vi "Gettag.vi"(0 "TagName":string="caca", 1 "XML":string="aaaa\n<caca noseque=nosecuanto>\nmás cosas\n</caca>\ndfsdf") -> (2 "AfterTag":string, 3 "InsideTag":string, 4 "BeforeTag":string="aaaa\n<caca noseque=nosecuanto>\nmás cosas\n</caca>\ndfsdf", 5 "Found?":bool)   [LabVIEW 2010]
panel:
  out "temp":string
  out "Inside":string
  out "N":i32=1
  # "This vi gets the contents of a tag and the strings after and before"
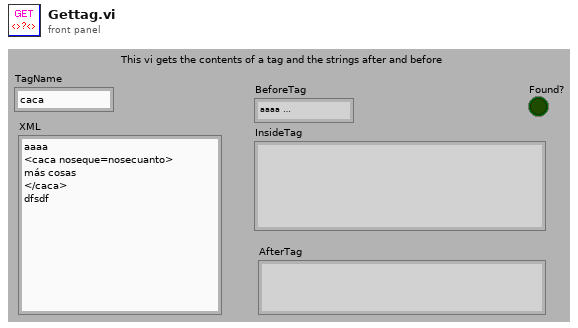
[diagram p1: front panel]
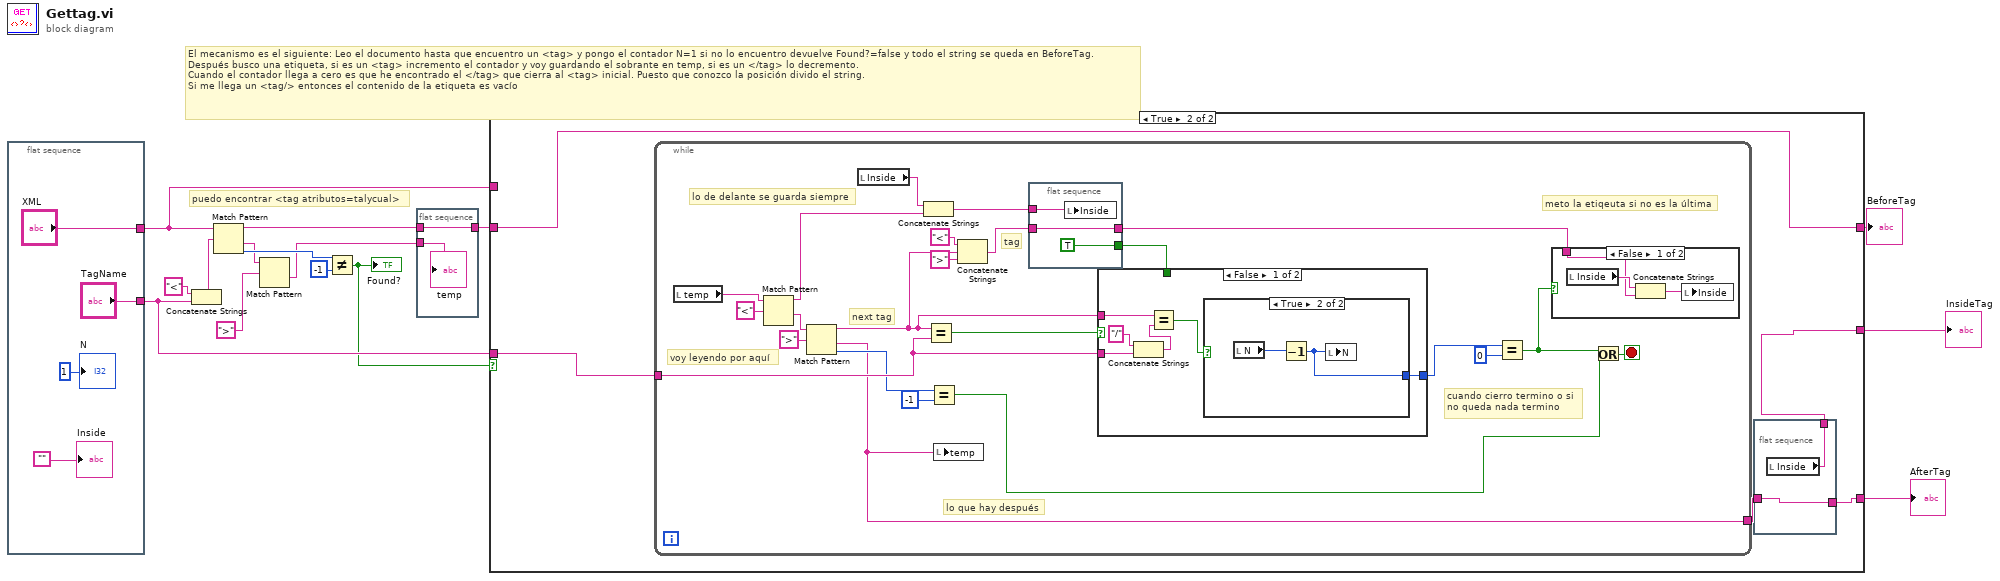
[diagram p0: block diagram]
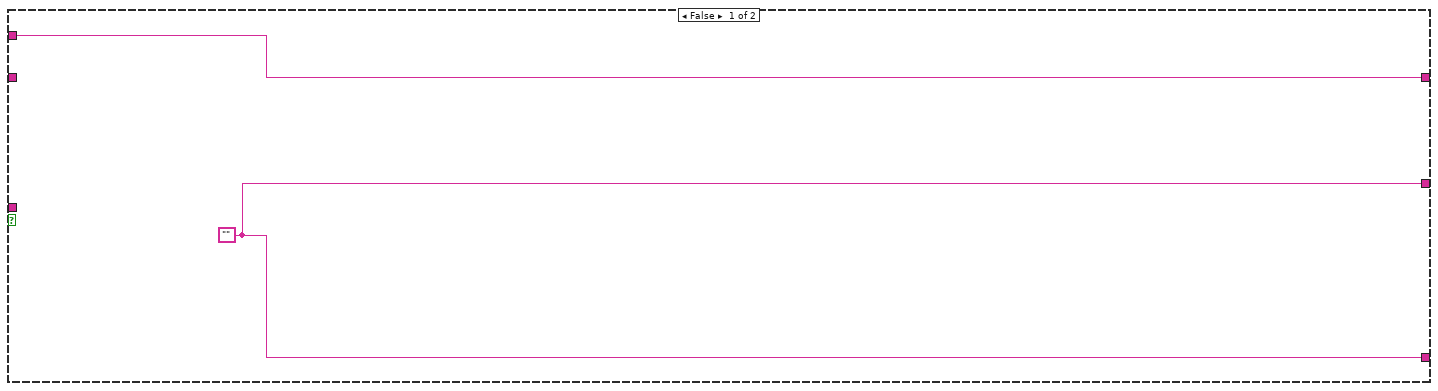
[diagram p2: hidden frame]
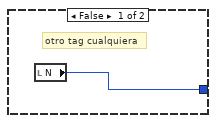
[diagram p4: hidden frame]
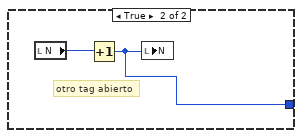
[diagram p5: hidden frame]
diagram:
  # "puedo encontrar <tag atributos=talycual>"
  # "El mecanismo es el siguiente: Leo el documento hasta que encuentro un <tag> y pongo el contador N=1 si no lo encuentro devuelve Found?=false y todo el string se queda en BeforeTag.\nDespués busco una etiqueta, si es un <tag> incremento el contador y voy guardando el sobrante en temp, si es un </tag> lo decremento.\nCuando el contador llega a cero es que he encontrado el </tag> que cierra al <tag> inicial. Puesto que conozco la posición divido el string.\nSi me llega un <tag/> entonces el contenido de la etiqueta es vacío"
  n1 = flat-sequence {
    tunnel: ["XML"] -> w11
    tunnel: ["TagName"] -> w7
    frame #0 {
      "N" <- 1
      "Inside" <- ""
    }
  }
  n2 = Concatenate Strings("<" ("string"), w7) -> (w8:string)
  n3 = Match Pattern(string=w11, regular expression=w8) -> (before substring=w5:string, after substring=w3:string, offset past match=w14:i32)  [unwired: 1 in, 1 out]
  n4 = Match Pattern(string=w3, regular expression=">" ("string")) -> (after substring=w1:string)  [unwired: 1 in, 3 out]
  n5 = Not Equal?(x=w14, y=-1) -> (x != y?=w6:bool)
  "Found?" <- w6
  n6 = flat-sequence {
    tunnel: w1 -> [w21]
    tunnel: w5 -> [w20]
    tunnel: [w20] -> w4
    frame #0 {
      "temp" <- w21
    }
  }
  n7 = case shown="True" w6 {
    tunnel: [w23 w27] -> w12
    tunnel: w4 -> [_ w27]
    tunnel: w11 -> [w23 _]
    tunnel: [w22 w24] -> w10
    tunnel: [w22 w26] -> w9
    tunnel: w7 -> [_ w28]
    frame False {
      w22 = ""
    }
    frame True {
      n8 = while {
        tunnel: w28 -> [w49]
        tunnel: [w39] -> w25
        stop <- w44 stop-if-true
        # "meto la etiqeuta si no es la última"
        # "lo de delante se guarda siempre"
        # "tag"
        # "lo que hay después"
        # "cuando cierro termino o si\nno queda nada termino"
        # "voy leyendo por aquí"
        # "next tag"
        n9 = local read "temp"() -> (w47:string)
        n10 = Match Pattern(string=w47, regular expression="<") -> (before substring=w36:string, after substring=w53:string)  [unwired: 1 in, 2 out]
        n11 = Match Pattern(string=w53, regular expression=">") -> (before substring=w42:string, after substring=w39:string, offset past match=w46:i32)  [unwired: 1 in, 1 out]
        n12 = local read "Inside"() -> (w37:string)
        n13 = Concatenate Strings(w37, w36) -> (w43:string)
        n14 = Equal?(x=w42, y=w49) -> (x = y?=w51:bool)
        n15 = Equal?(x=w46, y=-1) -> (x = y?=w34:bool)
        n16 = local write "temp"(w39) -> ()
        n17 = Concatenate Strings("<" ("before substring"), w42, ">" ("string")) -> (w38:string)
        n18 = flat-sequence {
          tunnel: w43 -> [w59]
          tunnel: w38 -> [w58]
          tunnel: [w58] -> w32
          tunnel: [TRUE] -> w31
          frame #0 {
            n19 = local write "Inside"(w59) -> ()
          }
        }
        n20 = case shown="False" w51 {
          tunnel: w42 -> [w65 _]
          tunnel: w49 -> [w64 _]
          tunnel: [w60 w69] -> w33
          tunnel: w31 -> [_ _]
          frame False {
            n21 = Concatenate Strings("/" ("string"), w64) -> (w63:string)
            n22 = Equal?(x=w65, y=w63) -> (x = y?=w61:bool)
            n23 = case shown="True" w61 {
              tunnel: [w66 w67] -> w60
              frame False {
                # "otro tag cualquiera"
                n24 = local read "N"() -> (w66:i32)
              }
              frame True {
                n25 = local read "N"() -> (w68:i32)
                n26 = Decrement(x=w68) -> (x-1=w67:i32)
                n27 = local write "N"(w67) -> ()
              }
            }
          }
          frame True {
            # "otro tag abierto"
            n28 = local read "N"() -> (w70:i32)
            n29 = Increment(x=w70) -> (x+1=w69:i32)
            n30 = local write "N"(w69) -> ()
          }
        }
        n31 = Equal?(x=w33, y=0) -> (x = y?=w35:bool)
        n32 = case shown="False" w35 {
          tunnel: w32 -> [w54 _]
          frame False {
            n33 = local read "Inside"() -> (w55:string)
            n34 = Concatenate Strings(w55, w54) -> (w56:string)
            n35 = local write "Inside"(w56) -> ()
          }
          frame True {
            # "el tag ya no se pone en inside"
          }
        }
        n36 = Or(x=w35, y=w34) -> (x .or. y?=w44:bool)
      }
      n37 = flat-sequence {
        tunnel: [w30] -> w26
        tunnel: w25 -> [w30]
        tunnel: [w29] -> w24
        frame #0 {
          n38 = local read "Inside"() -> (w29:string)
        }
      }
    }
  }
  "AfterTag" <- w9
  "BeforeTag" <- w12
  "InsideTag" <- w10
